vi "Spectrograph_getSample_timestamp.vi"(8 "error in (no error)":errorcluster, 11 "timestamp_Ctl":T1) -> (0 "error out":errorcluster, 2 "function return":i32, 3 "timestamp_Ctl out":T1)   [LabVIEW 2016, in "SALLV_Spectrograph.lvlib"]
doc: "int Spectrograph_shm_getSample_timestampLV(Spectrograph_timestampLV *timestamp_Ctl );"
uses:
  SALLV_Spectrograph.lvlib
  DataTypes/timestamp.ctl
  SALLV_Spectrograph.so
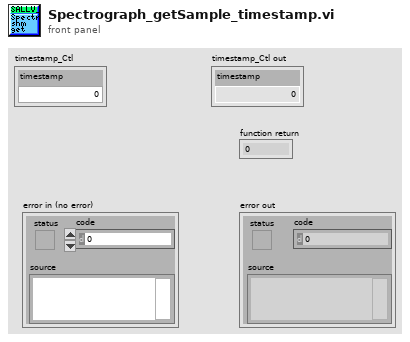
[diagram p1: front panel]
types:
  T1 = typedef "SALLV_Spectrograph.lvlib/timestamp.ctl" = cluster{"timestamp":dbl}
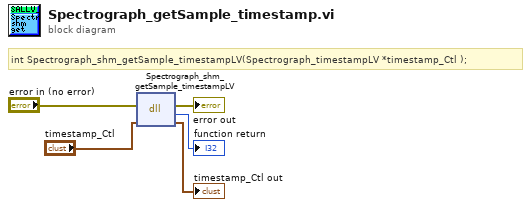
[diagram p0: block diagram]
diagram:
  # "int Spectrograph_shm_getSample_timestampLV(Spectrograph_timestampLV *timestamp_Ctl );"
  n1 = dll-call lib="home/harini/TCS/SALLV_Spectrograph/SALLV_Spectrograph.*" fn="Spectrograph_shm_getSample_timestampLV"(error in="error in (no error)", "timestamp_Ctl"="timestamp_Ctl") -> (error out=→"error out":errorcluster, →"function return":i32, "timestamp_Ctl"=→"timestamp_Ctl out":T1)  [unwired: 2 in, 1 out]
